vi "GEA2 Serial Get CRC2.vi"(8 "Error In":errorcluster, 9 "Current Read Index":i32, 10 "CRCRead":u8[](array[numeric]), 11 "ReadArray":u8[](array[numeric])) -> (0 "Error Out":errorcluster, 2 "CRC Read":u8[](array[numeric]), 3 "Current Read Index":i32)   [LabVIEW 2014]
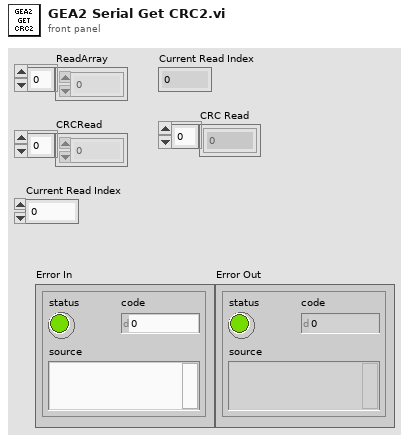
[diagram p1: front panel]
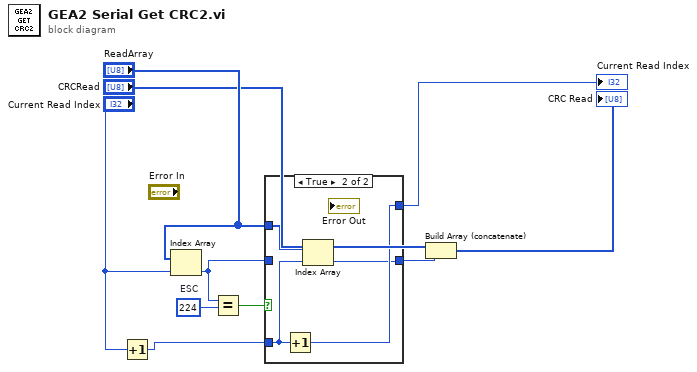
[diagram p0: block diagram]
diagram:
  w1 = u8 224  # ESC
  n1 = Increment(x="Current Read Index") -> (x+1=w8:i32)
  n2 = Index Array(array="ReadArray", index="Current Read Index") -> (element=w10:u8)
  n3 = Equal?(x=w10, y=w1) -> (x = y?=w2:bool)
  n4 = case shown="True" w2 {
    tunnel: [w11 w13] -> w4
    tunnel: [w12 w16] -> w3
    tunnel: "ReadArray" -> [_ w15]
    tunnel: w8 -> [w12 w14]
    tunnel: w10 -> [w11 _]
    frame False {
    }
    frame True {
      n5 = Increment(x=w14) -> (x+1=w16:i32)
      n6 = Index Array(array=w15, index=w14) -> (element=w13:u8)
    }
  }
  "Current Read Index" <- w3
  n7 = Build Array (concatenate)("CRCRead", w4) -> (→"CRC Read":u8[])
